vi "Converti_ dati Elettrotest60A.vi"(11 "String in":string) -> (0 "libero1 2":bool, 1 "libero1":bool, 2 "Check last 2bit(T=OK)":bool, 3 "Converted":dbl, 4 "FS 2":T1={"Resistenza1"=2.0, "Resistenza2"=2.0, "RESISTENZA"=2.0})   [LabVIEW 2019]
panel:
  out "Boolean array":bool[](array[boolean])
  out "element":bool
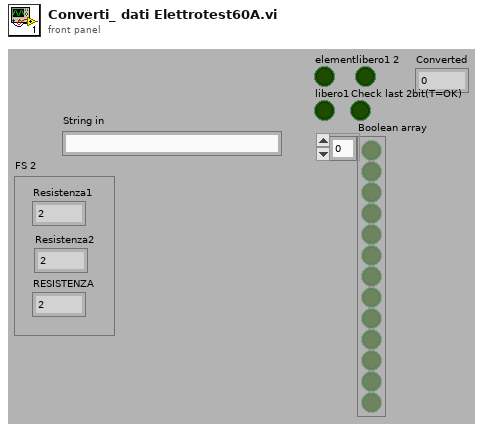
[diagram p1: front panel]
types:
  T1 = cluster{"Resistenza1":dbl, "Resistenza2":dbl, "RESISTENZA":dbl}
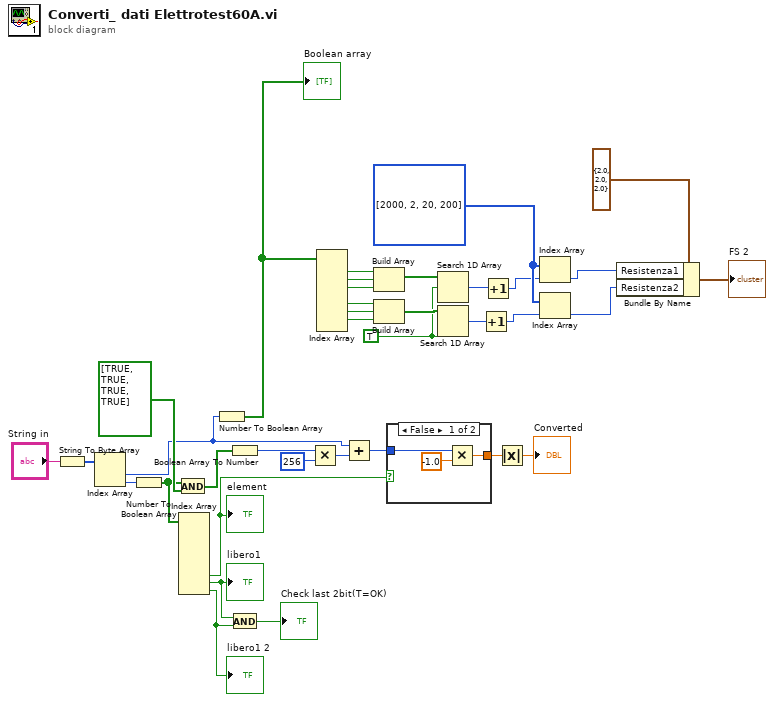
[diagram p0: block diagram]
diagram:
  w5 = TRUE ("element")
  w10 = i32[] [2000, 2, 20, 200]
  n1 = String To Byte Array(string="String in") -> (unsigned byte array=w35:u8[])
  n2 = Index Array(array=w35) -> (element #1=w21:u8, element #2=w8:u8)  [unwired: 2 in]
  n3 = Number To Boolean Array(number=w8) -> (Boolean array=w30:bool[])
  n4 = And(x=w30, y=bool[] [TRUE, TRUE, TRUE, TRUE]) -> (x .and. y?=w33:bool[])
  n5 = Index Array(array=w30) -> (element #6=w29:bool, element #7=w27:bool, element #8=w26:bool)  [unwired: 8 in, 5 out]
  "element" <- w29
  "libero1" <- w27
  "libero1 2" <- w26
  n6 = Number To Boolean Array(number=w21) -> (Boolean array=w20:bool[])
  "Boolean array" <- w20
  n7 = Boolean Array To Number(Boolean array=w33) -> (number=w22:u32)
  n8 = And(x=w27, y=w26) -> (x .and. y?=→"Check last 2bit(T=OK)":bool)
  n9 = Multiply(x=w22, y=u32 256) -> (x*y=w31:u32)
  n10 = Index Array(array=w20) -> (element #1=w19:bool, element #2=w18:bool, element #3=w17:bool, element #5=w16:bool, element #6=w15:bool, element #7=w14:bool)  [unwired: 8 in, 2 out]
  n11 = Add(x=w21, y=w31) -> (x+y=w28:u32)
  n12 = Build Array(w19, w18, w17) -> (w7:bool[])
  n13 = Build Array(w16, w15, w14) -> (w6:bool[])
  n14 = case shown="False" w29 {
    tunnel: w28 -> [w39 w40]
    tunnel: [w37 w40] -> w24
    frame False {
      n15 = Multiply(x=w39, y=-1.0) -> (x*y=w37:dbl)
    }
    frame True {
    }
  }
  n16 = Search 1D Array(1D array=w7, element=w5) -> (index of element=w4:i32)  [unwired: 1 in]
  n17 = Search 1D Array(1D array=w6, element=w5) -> (index of element=w2:i32)  [unwired: 1 in]
  n18 = Increment(x=w2) -> (x+1=w1:i32)
  n19 = Increment(x=w4) -> (x+1=w3:i32)
  n20 = Absolute Value(x=w24) -> (abs(x)=→"Converted":dbl)
  n21 = Index Array(array=w10, index=w3) -> (element=w11:i32)
  n22 = Index Array(array=w10, index=w1) -> (element=w9:i32)
  n23 = Bundle By Name(cluster=T1 {"Resistenza1"=2.0, "Resistenza2"=2.0, "RESISTENZA"=2.0} ("FS 2"), "Resistenza1"=w11, "Resistenza2"=w9) -> (→"FS 2":T1)
